vi "Scan Initilize_without Accurate Measure.vi"(8 "error in (no error)":errorcluster, 9 "Current Setting":u8[](array[numeric]), 10 "Channel Count":i32, 11 "VISA Refnum in":refnum<visa-resource-name>) -> (0 "error out":errorcluster, 1 "N channel number":i32, 2 "P channel number":i32, 3 "VISA Refnum out":refnum<visa-resource-name>, 5 "Current Channel":string[](array[string]))   [LabVIEW 2023]
uses:
  <instrlib>/Agilent 3446X Series/Agilent 3446X Series.lvlib
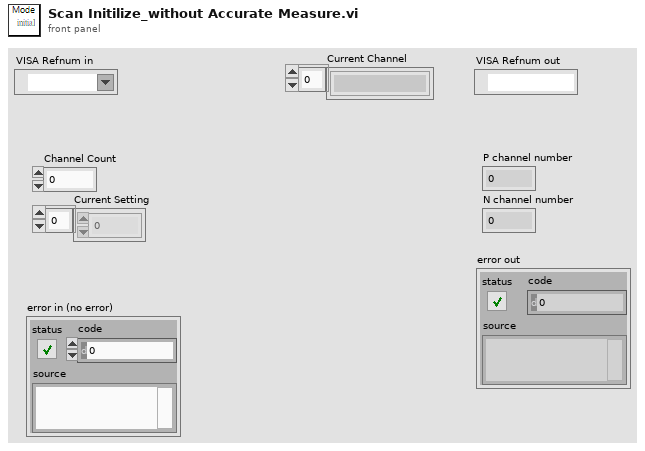
[diagram p1: front panel]
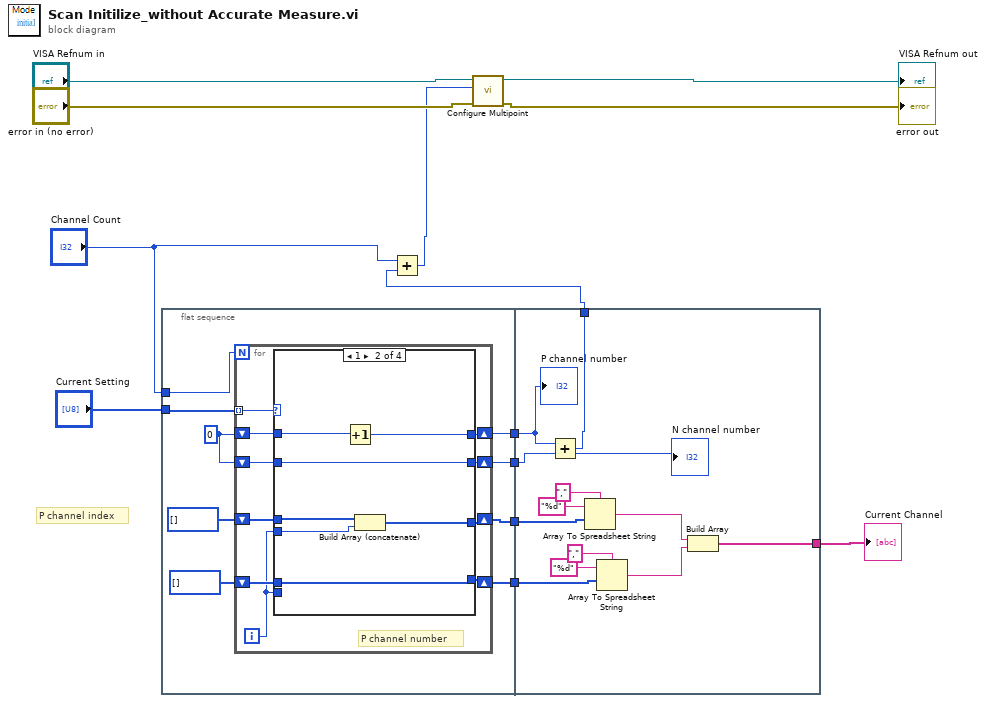
[diagram p0: block diagram]
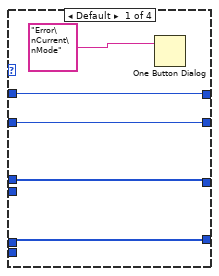
[diagram p2: hidden frame]
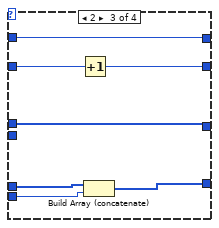
[diagram p3: hidden frame]
diagram:
  # "P channel index"
  # "P channel number"
  n1 = flat-sequence {
    tunnel: "Channel Count" -> [w22]
    tunnel: "Current Setting" -> [w21]
    tunnel: [w19] -> w9
    tunnel: [w18] -> w8
    tunnel: [w15] -> w7
    tunnel: [w14] -> w6
    tunnel: w9 -> [w67]
    tunnel: w8 -> [w66]
    tunnel: [w65] -> w2
    tunnel: w7 -> [w62]
    tunnel: w6 -> [w59]
    tunnel: [w56] -> w3
    frame #0 {
      w20 = 0 ("P_current_count")
      n2 = for {
        N: w22 -> [_]
        tunnel: w21 -> [w32] mode=indexing
        shift-right: [w30] -> w19
        shift-left: w20 -> [w31]
        shift-right: [w28] -> w18
        shift-left: w20 -> [w29]
        shift-right: [w26] -> w15
        shift-left: i32[] [] -> [w27]
        shift-right: [w24] -> w14
        shift-left: i32[] [] -> [w25]
        i -> [w23]
        n3 = case shown="1" w32 {
          tunnel: w31 -> [w36 w44 w49 w55]
          tunnel: [w36 w43 w49 w55] -> w30
          tunnel: w29 -> [w35 w42 w51 w54]
          tunnel: [w35 w42 w50 w54] -> w28
          tunnel: w27 -> [w33 w41 w45 w53]
          tunnel: w23 -> [_ w40 _ _]
          tunnel: [w33 w39 w45 w53] -> w26
          tunnel: w25 -> [w34 w38 w48 w52]
          tunnel: [w34 w38 w47 w52] -> w24
          tunnel: w23 -> [_ _ w46 _]
          frame Default {
            n4 = One Button Dialog(message="Error\nCurrent\nMode" ("error source (\" \")")) -> ()  [unwired: 1 in, 1 out]
          }
          frame 1 {
            n5 = Increment(x=w44) -> (x+1=w43:i32)
            n6 = Build Array (concatenate)(w41, w40) -> (w39:i32[])
          }
          frame 2 {
            n7 = Increment(x=w51) -> (x+1=w50:i32)
            n8 = Build Array (concatenate)(w48, w46) -> (w47:i32[])
          }
          frame 0 {
          }
        }
      }
    }
    frame #1 {
      n9 = Add(x=w67, y=w66) -> (x+y=w65:i32)
      n10 = Array To Spreadsheet String(delimiter (Tab)=",", array=w62, 3:"%d" ("format string")) -> (spreadsheet string=w58:string)
      n11 = Array To Spreadsheet String(delimiter (Tab)=",", array=w59, 3:"%d" ("format string")) -> (spreadsheet string=w57:string)
      n12 = Build Array(w58, w57) -> (w56:string[])
      "P channel number" <- w67
      "N channel number" <- w66
    }
  }
  n13 = Add(x="Channel Count", y=w2) -> (x+y=w1:i32)
  n14 = call <instrlib>:"Configure Multipoint.vi"("error in (no error)"="error in (no error)", "Trigger Count (1)"=w1, "VISA resource name"="VISA Refnum in") -> ("error out"=→"error out":errorcluster, "VISA resource name out"=→"VISA Refnum out":refnum<visa-resource-name>)  [unwired: 4 in, 3 out]
  "Current Channel" <- w3
